vi "CreateNewWizard_IncludeItem.vi"(11 "Wizard":T1) -> (3 "Include me":bool)   [LabVIEW 2020, in "Add Actor Interface.lvlib"]
uses:
  Add Actor Interface.lvlib
  <resource>/Framework/Providers/API/ItemRef.ctl
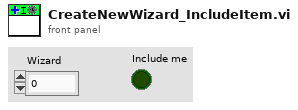
[diagram p1: front panel]
types:
  T1 = typedef "ItemRef.ctl" = u64
  T2 = typedef "mxLvNIIM.ctl" = cluster{"Item URL":string, "Item ID":string, "Item Index":i32, "Specific Type":string}
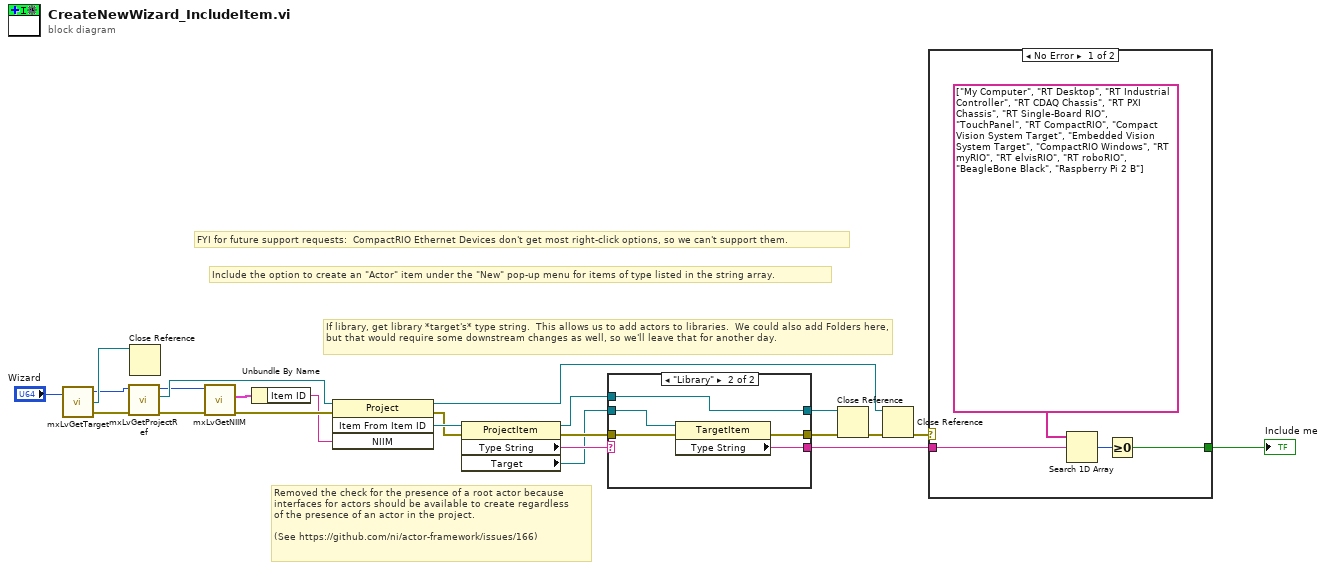
[diagram p0: block diagram]
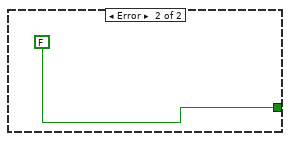
[diagram p3: hidden frame]
diagram:
  # "Removed the check for the presence of a root actor because\ninterfaces for actors should be available to create regardless\nof the presence of an actor in the project.\n\n(See https://github.com/ni/actor-framework/issues/166)"
  # "FYI for future support requests:  CompactRIO Ethernet Devices don't get most right-click options, so we can't support them."
  # "If library, get library *target's* type string.  This allows us to add actors to libraries.  We could also add Folders here, but that would require some downstream changes as well, so we'll leave that for another day."
  # "Include the option to create an \"Actor\" item under the \"New\" pop-up menu for items of type listed in the string array."
  n1 = call <resource>:"mxLvGetTarget.vi"("Item"="Wizard") -> ("Item"=w16:T1, "Target"=w18:refnum<vi>, "error out"=w17:errorcluster)  [unwired: 1 in]
  n2 = call <resource>:"mxLvGetProjectRef.vi"("error in"=w17, "Item"=w16) -> ("error out"=w23:errorcluster, "Project Refnum"=w19:refnum<vi>, "Item"=w14:T1)  [unwired: 7 in]
  n3 = Close Reference(reference=w18) -> ()  [unwired: 1 in, 1 out]
  n4 = call <resource>:"mxLvGetNIIM.vi"("error in"=w23, "Item"=w14) -> ("error out"=w21:errorcluster, "NIIM"=w20:T2)  [unwired: 7 in, 1 out]
  n5 = Unbundle By Name(w20) -> ("Item ID"=w4:string)
  n6 = invoke class="Project" method="Item From Item ID"(reference=w19, error in=w21, "NIIM"=w4) -> (reference out=w7:refnum<vi>, error out=w12:errorcluster, "GetItemFromNIIM"=w22:refnum<vi>)  [unwired: 1 in, 1 out]
  n7 = property class="ProjectItem"(reference=w22, error in=w12) -> (reference out=w13:refnum<vi>, error out=w3:errorcluster, "Type String"=w6:string, "Target"=w2:refnum<vi>)
  n8 = case shown="\"Library\"" w6 {
    selector: w6 -> [w24 _]
    tunnel: w3 -> [w25 w27]
    tunnel: w13 -> [w26 w28]
    tunnel: [w24 w31] -> w5
    tunnel: [w25 w30] -> w11
    tunnel: [w26 w28] -> w10
    tunnel: w2 -> [_ w29]
    frame Default {
    }
    frame "Library" {
      n9 = property class="TargetItem"(reference=w29, error in=w27) -> (error out=w30:errorcluster, "Type String"=w31:string)  [unwired: 1 out]
    }
  }
  n10 = Close Reference(reference=w10, error in (no error)=w11) -> (error out=w9:errorcluster)
  n11 = Close Reference(reference=w7, error in (no error)=w9) -> (error out=w8:errorcluster)
  n12 = case shown="No Error" w8 {
    tunnel: w5 -> [w35 _]
    tunnel: [w33 FALSE] -> w1
    frame No Error {
      n13 = Search 1D Array(1D array=string[] ["My Computer", "RT Desktop", "RT Industrial Controller", "RT CDAQ Chassis", "RT PXI Chassis", "RT Single-Board RIO", "TouchPanel", "RT CompactRIO", "Compact Vision System Target", "Embedded Vision System Target", "CompactRIO Windows", "RT myRIO", "RT elvisRIO", "RT roboRIO", "BeagleBone Black", "Raspberry Pi 2 B"] ("Array"), element=w35) -> (index of element=w34:i32)  [unwired: 1 in]
      n14 = Greater Or Equal To 0?(x=w34) -> (x >= 0?=w33:bool)
    }
    frame Error {
    }
  }
  "Include me" <- w1
